vi "test_libssh2_session_hostkey.vi"() -> ()   [LabVIEW 2013, in "libssh2_integration_tests.lvlib"]
uses:
  libssh2_integration_tests.lvlib
  <vilib>/addons/_JKI Toolkits/Caraya/classes/Test/Test.lvclass
  libssh2/libssh2.lvlib
  <vilib>/addons/_JKI Toolkits/Caraya/classes/Assert/Assert.lvclass
panel:
  out "error out":errorcluster
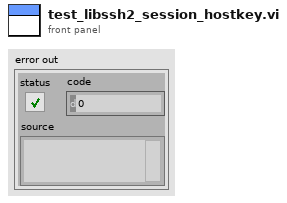
[diagram p1: front panel]
types:
  T1 = typedef "libssh2.lvlib/Session Refnum.ctl" = refnum<k1>
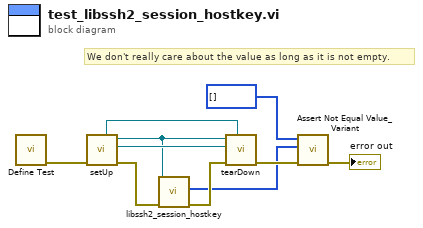
[diagram p0: block diagram]
diagram:
  # "We don't really care about the value as long as it is not empty."
  n1 = call <vilib>:"Define Test.vi"() -> ("error out"=w10:errorcluster)  [unwired: 10 in, 1 out]
  n2 = call "setUp.vi"("error in (no error)"=w10) -> ("error out"=w5:errorcluster, "connection ID"=w9:refnum<k5>, "session"=w7:T1, "fixture"=w8:refnum<class "Server Fixture.lvclass">)  [unwired: 7 in]
  n3 = call "libssh2_session_hostkey.vi"("error in (no error)"=w5, "session"=w7) -> ("error out"=w6:errorcluster, "hostkey"=w1:u8[])  [unwired: 7 in, 1 out]
  n4 = call "tearDown.vi"("fixture"=w8, "error in (no error)"=w6, "connection ID"=w9, "session"=w7) -> ("error out"=w4:errorcluster)  [unwired: 7 in]
  n5 = call <vilib>:"Assert Not Equal Value_Variant.vi"("error in (no error)"=w4, "Y"=w1, "X"=u8[] []) -> ("error out"=→"error out":errorcluster)  [unwired: 7 in, 1 out]
